vi "Real Coordinates convert.vi"(9 "Mode":T1(ring), 10 "Coordinates(X,Y)":cluster{"X":dbl, "Y":dbl}, 11 "Overlay Setting":T2) -> (3 "Real Coordinates(X,Y)":cluster{dbl, dbl})   [LabVIEW 2015]
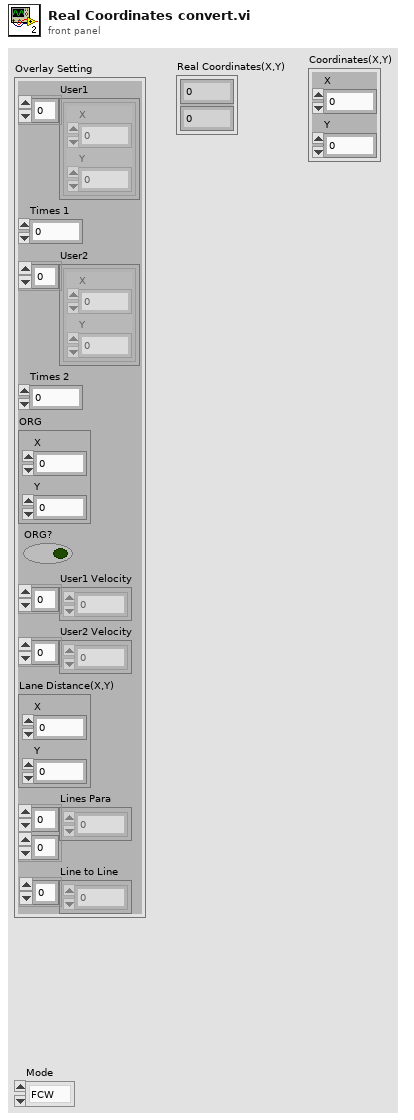
[diagram p1: front panel]
types:
  T1 = enum16{"FCW", "BSD(Right)", "BSD(Left)", "RCTA(Right)", "RCTA(Left)", "DOW(Right)", "DOW(Left)"}
  T2 = cluster{"User1":cluster{"X":dbl, "Y":dbl}[], "Times 1":i32, "User2":cluster{"X":dbl, "Y":dbl}[], "Times 2":i32, "ORG":cluster{"X":dbl, "Y":dbl}, "ORG?":bool, "User1 Velocity":dbl[], "User2 Velocity":dbl[], "Lane Distance(X,Y)":cluster{"X":dbl, "Y":dbl}, "Lines Para":dbl[][], "Line to Line":dbl[]}
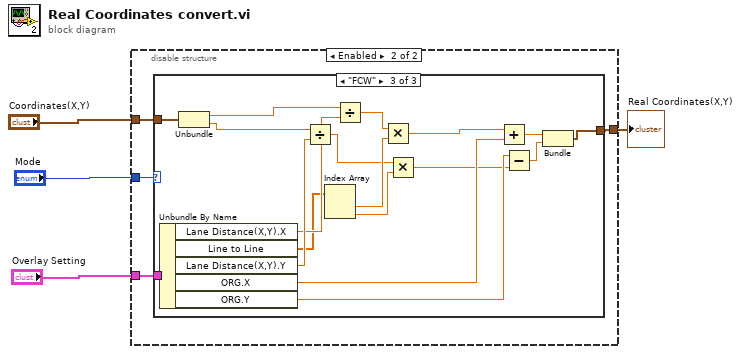
[diagram p0: block diagram]
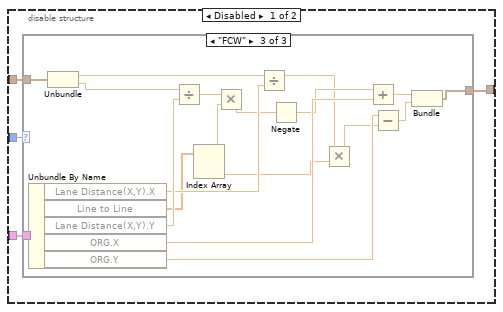
[diagram p2: hidden frame]
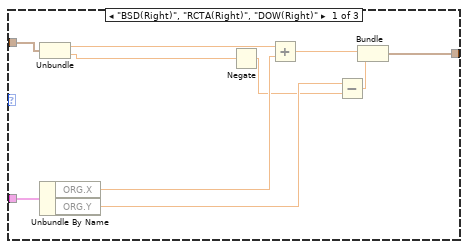
[diagram p3: hidden frame]
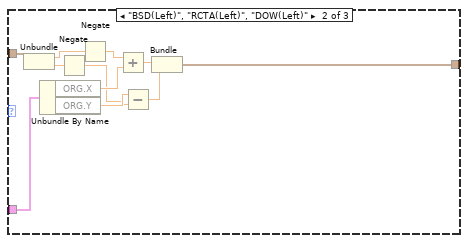
[diagram p4: hidden frame]
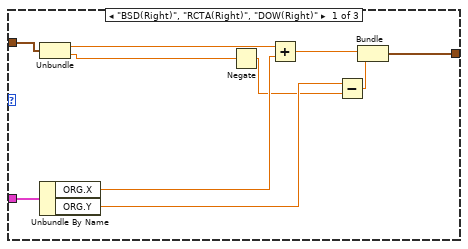
[diagram p5: hidden frame]
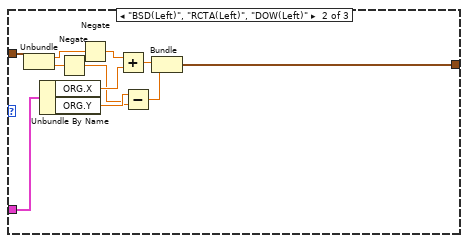
[diagram p6: hidden frame]
diagram:
  n1 = disable-structure shown="Enabled" {
    disable-tunnel: [w8 w49] -> w4
    disable-tunnel: "Overlay Setting" -> [w7 w50]
    disable-tunnel: "Coordinates(X,Y)" -> [w6 w52]
    disable-tunnel: "Mode" -> [w5 w51]
    frame Disabled {
      n2 = case shown="\"FCW\"" w5 {
        tunnel: w6 -> [w17 w28 w47]
        tunnel: w7 -> [w18 w29 w48]
        tunnel: [w13 w24 w45] -> w8
        frame "BSD(Right)", "RCTA(Right)", "DOW(Right)" {
          n3 = Unbundle(w17) -> ("X"=w15:dbl, "Y"=w10:dbl)
          n4 = Unbundle By Name(w18) -> ("ORG.X"=w16:dbl, "ORG.Y"=w11:dbl)
          n5 = Negate(x=w10) -> (-x=w9:dbl)
          n6 = Add(x=w15, y=w16) -> (x+y=w14:dbl)
          n7 = Subtract(x=w11, y=w9) -> (x-y=w12:dbl)
          n8 = Bundle(w14, w12) -> (w13:cluster{dbl, dbl})  [unwired: 1 in]
        }
        frame "BSD(Left)", "RCTA(Left)", "DOW(Left)" {
          n9 = Unbundle(w28) -> ("X"=w26:dbl, "Y"=w21:dbl)
          n10 = Unbundle By Name(w29) -> ("ORG.X"=w27:dbl, "ORG.Y"=w22:dbl)
          n11 = Negate(x=w21) -> (-x=w19:dbl)
          n12 = Negate(x=w26) -> (-x=w20:dbl)
          n13 = Add(x=w20, y=w27) -> (x+y=w25:dbl)
          n14 = Subtract(x=w22, y=w19) -> (x-y=w23:dbl)
          n15 = Bundle(w25, w23) -> (w24:cluster{dbl, dbl})  [unwired: 1 in]
        }
        frame "FCW" {
          n16 = Unbundle By Name(w48) -> ("Lane Distance(X,Y).X"=w38:dbl, "Line to Line"=w35:dbl[], "Lane Distance(X,Y).Y"=w40:dbl, "ORG.X"=w44:dbl, "ORG.Y"=w43:dbl)
          n17 = Unbundle(w47) -> ("X"=w30:dbl, "Y"=w31:dbl)
          n18 = Divide(x=w31, y=w40) -> (x/y=w36:dbl)
          n19 = Index Array(array=w35) -> (element #1=w33:dbl, element #2=w32:dbl)  [unwired: 2 in]
          n20 = Multiply(x=w36, y=w33) -> (x*y=w37:dbl)
          n21 = Divide(x=w30, y=w38) -> (x/y=w39:dbl)
          n22 = Negate(x=w37) -> (-x=w41:dbl)
          n23 = Multiply(x=w39, y=w32) -> (x*y=w34:dbl)
          n24 = Add(x=w41, y=w44) -> (x+y=w46:dbl)
          n25 = Subtract(x=w43, y=w34) -> (x-y=w42:dbl)
          n26 = Bundle(w46, w42) -> (w45:cluster{dbl, dbl})  [unwired: 1 in]
        }
      }
    }
    frame Enabled {
      n27 = case shown="\"FCW\"" w51 {
        tunnel: w52 -> [w61 w72 w90]
        tunnel: w50 -> [w62 w73 w91]
        tunnel: [w57 w68 w88] -> w49
        frame "BSD(Right)", "RCTA(Right)", "DOW(Right)" {
          n28 = Unbundle(w61) -> ("X"=w59:dbl, "Y"=w54:dbl)
          n29 = Unbundle By Name(w62) -> ("ORG.X"=w60:dbl, "ORG.Y"=w55:dbl)
          n30 = Negate(x=w54) -> (-x=w53:dbl)
          n31 = Add(x=w59, y=w60) -> (x+y=w58:dbl)
          n32 = Subtract(x=w55, y=w53) -> (x-y=w56:dbl)
          n33 = Bundle(w58, w56) -> (w57:cluster{dbl, dbl})  [unwired: 1 in]
        }
        frame "BSD(Left)", "RCTA(Left)", "DOW(Left)" {
          n34 = Unbundle(w72) -> ("X"=w70:dbl, "Y"=w65:dbl)
          n35 = Unbundle By Name(w73) -> ("ORG.X"=w71:dbl, "ORG.Y"=w66:dbl)
          n36 = Negate(x=w65) -> (-x=w63:dbl)
          n37 = Negate(x=w70) -> (-x=w64:dbl)
          n38 = Add(x=w64, y=w71) -> (x+y=w69:dbl)
          n39 = Subtract(x=w66, y=w63) -> (x-y=w67:dbl)
          n40 = Bundle(w69, w67) -> (w68:cluster{dbl, dbl})  [unwired: 1 in]
        }
        frame "FCW" {
          n41 = Unbundle By Name(w91) -> ("Lane Distance(X,Y).X"=w83:dbl, "Line to Line"=w82:dbl[], "Lane Distance(X,Y).Y"=w84:dbl, "ORG.X"=w87:dbl, "ORG.Y"=w86:dbl)
          n42 = Unbundle(w90) -> ("X"=w80:dbl, "Y"=w81:dbl)
          n43 = Divide(x=w81, y=w84) -> (x/y=w77:dbl)
          n44 = Index Array(array=w82) -> (element #1=w78:dbl, element #2=w76:dbl)  [unwired: 2 in]
          n45 = Divide(x=w80, y=w83) -> (x/y=w79:dbl)
          n46 = Multiply(x=w79, y=w78) -> (x*y=w74:dbl)
          n47 = Multiply(x=w77, y=w76) -> (x*y=w75:dbl)
          n48 = Add(x=w74, y=w87) -> (x+y=w89:dbl)
          n49 = Subtract(x=w86, y=w75) -> (x-y=w85:dbl)
          n50 = Bundle(w89, w85) -> (w88:cluster{dbl, dbl})  [unwired: 1 in]
        }
      }
    }
  }
  "Real Coordinates(X,Y)" <- w4
